vi "Keithley 6514 Block Read.vi"(0 "Resource In":refnum<visa-resource-name>, 1 "Check For SCPI Errors? (T)":bool=TRUE, 11 "error in (no error)":T1, 12 "Timeout (5000 msecs)":u32=5000) -> (4 "Resource Out (dupl)":refnum<visa-resource-name>, 6 "Num Meas":i32 min=0 max=2500, 8 "Test Data":sgl[][](array[numeric]) format="%^.4e", 10 "Data Elements":string, 15 "error out":T1)   [LabVIEW 2014, in "KE6514Driver.lvlib"]
doc: "This VI is used to perform a block read with the 6514. The VI will return the actual number of points that was read, the data format used for the data transfer, the data elements returned and the actual data which is stored in a LabVIEW array.\n\nNOTE: THIS VI WILL NOT EXECUTE CORRECTLY IF THE GPIB TIMEOUT FUNCTION IS NOT LONG ENOUGH. IF YOUR OPERATION TAKES LONGER THAN THE TIMEOUT PERIOD, INCORRECT OPERATION WILL OCCUR. THE VI SENDS OUT THE SCPI 'READ?' COMMAND. WHEN THIS COMMAND IS SENT OVER THE BUS, THE 24XX PERFORMS A SCPI 'INIT' FUNCTION WHICH INITIALIZES THE TRIGGERING AND BEGINS TAKING MEASUREMENTS. WHEN ALL MEASUREMENTS HAVE BEEN TAKEN, THE DATA IS RETURNED. AGAIN, IF THE TIMEOUT IS SMALLER THAN THE TIME IT TAKES TO COMPLETE THE MEASUREMENT OPERATIONS, INCORRECT RESULTS WILL OCCUR. IT IS RECOMMENDED TO SET THE TIMEOUT TO A LARGE VALUE TO PREVENT ERRORS.\n\nDEFAULTS: \nGPIB Address = 14\n\nMeasurements:\nReturned by instrument. Not user settable. 1 to 2500.\n\nData Format: \nReturned by instrument. Not user settable. Format returned is 'ASC' for ASCII and 'SRE' for Single Precision Real.\n\nData Elements:\nReturned by instrument. Not user settable. The order in which the elements are returned reflects the order in which each sample point is presented in the array. Main order is:\nREAD,TIME, STAT\n\nwhere:\nREAD = Reading\nTIME = Time Stamp\nSTAT = Status (Refer to Instrument Users manual to decode the status).\n\nTest Data:\nThis is an array where the sample data is placed after transfer over the bus. The order for which the data is presented appears in the 'Data Elements' indicator. Maximum number of data points returned is 2500."
uses:
  KE6514Driver.lvlib
panel:
  out "Max Num Bytes To Read For ASCII":i32
  out "Num Bytes To Read For Binary":i32
  out "Data Format":string
  # "NOTE: YOU MUST HAVE EXECUTED THE\n'BLOCK READ SETUP' VI AT LEAST ONCE\nPRIOR TO USING THIS VI."
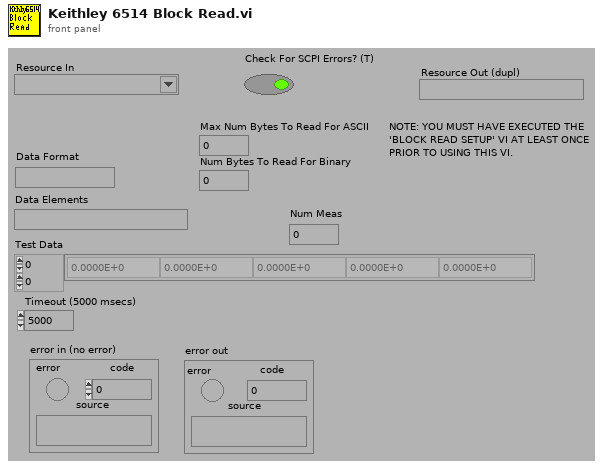
[diagram p1: front panel]
types:
  T1 = cluster{"error":bool, "code":i32, "source":string}
  T2 = enum16{"big-endian, network order", "native, host order", "little-endian"}
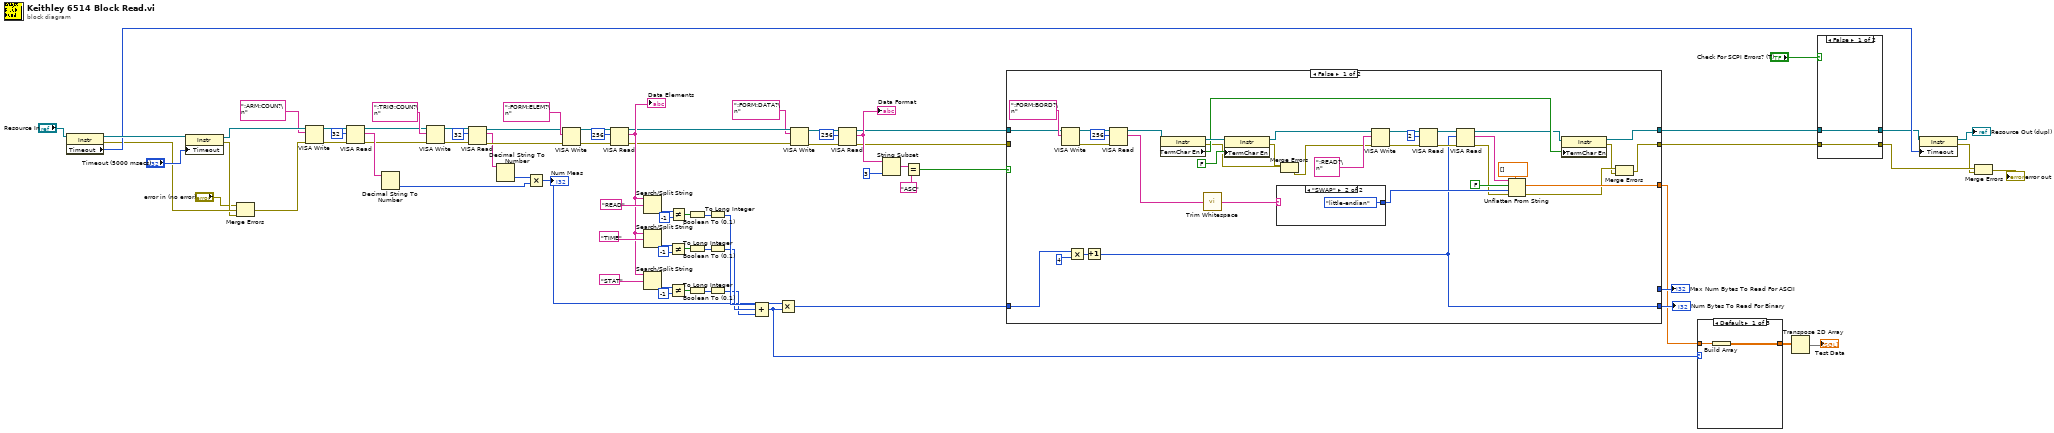
[diagram p0: block diagram]
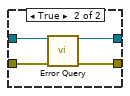
[diagram p2: hidden frame]
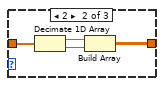
[diagram p3: hidden frame]
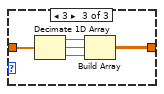
[diagram p4: hidden frame]
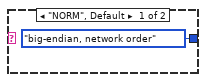
[diagram p5: hidden frame]
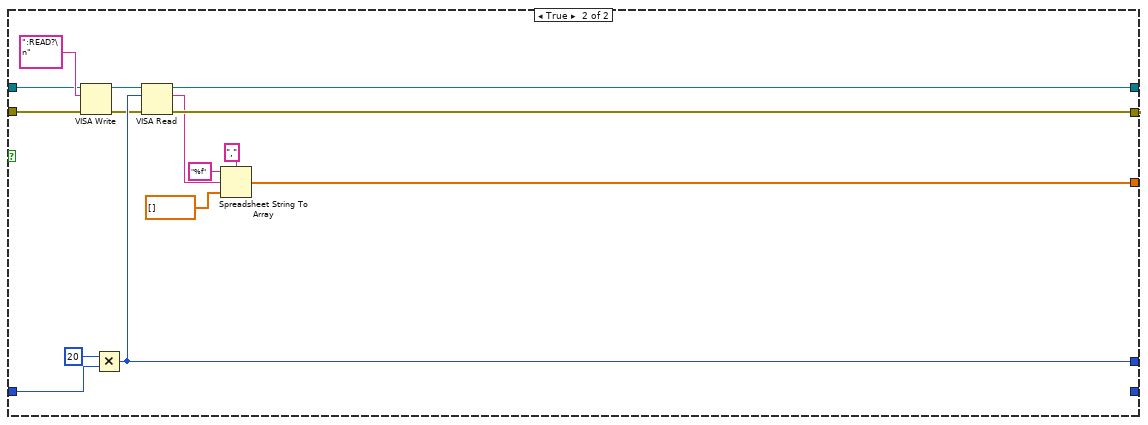
[diagram p6: hidden frame]
diagram:
  n1 = property class="Instr"(reference="Resource In") -> (reference out=w77:refnum<visa-resource-name>, error out=w4:errorcluster, "Timeout"=w13:u32)  [unwired: 1 in]
  n2 = property class="Instr"(reference=w77, "Timeout"="Timeout (5000 msecs)") -> (reference out=w75:refnum<visa-resource-name>, error out=w3:errorcluster)  [unwired: 1 in]
  n3 = Merge Errors("error in (no error)", w4, w3) -> (w1:errorcluster)
  n4 = VISA Write(VISA resource name=w75, write buffer=":ARM:COUN?\n", error in (no error)=w1) -> (VISA resource name out=w73:refnum<visa-resource-name>, error out=w71:errorcluster)  [unwired: 1 out]
  n5 = VISA Read(VISA resource name=w73, byte count=u32 32, error in (no error)=w71) -> (VISA resource name out=w65:refnum<visa-resource-name>, read buffer=w70:string, error out=w64:errorcluster)  [unwired: 1 out]
  n6 = Decimal String To Number(string=w70) -> (number=w63:i32)  [unwired: 2 in, 1 out]
  n7 = VISA Write(VISA resource name=w65, write buffer=":TRIG:COUN?\n", error in (no error)=w64) -> (VISA resource name out=w68:refnum<visa-resource-name>, error out=w66:errorcluster)  [unwired: 1 out]
  n8 = VISA Read(VISA resource name=w68, byte count=u32 32, error in (no error)=w66) -> (VISA resource name out=w58:refnum<visa-resource-name>, read buffer=w37:string, error out=w57:errorcluster)  [unwired: 1 out]
  n9 = Decimal String To Number(string=w37) -> (number=w36:i32)  [unwired: 2 in, 1 out]
  n10 = Multiply(x=w36, y=w63) -> (x*y=w24:i32)
  "Num Meas" <- w24
  n11 = VISA Write(VISA resource name=w58, write buffer=":FORM:ELEM?\n", error in (no error)=w57) -> (VISA resource name out=w61:refnum<visa-resource-name>, error out=w60:errorcluster)  [unwired: 1 out]
  n12 = VISA Read(VISA resource name=w61, byte count=u32 256, error in (no error)=w60) -> (VISA resource name out=w29:refnum<visa-resource-name>, read buffer=w38:string, error out=w27:errorcluster)  [unwired: 1 out]
  "Data Elements" <- w38
  n13 = Search/Split String(string=w38, search string/char (-)="TIME") -> (offset of match=w53:i32)  [unwired: 1 in, 2 out]
  n14 = Search/Split String(string=w38, search string/char (-)="STAT") -> (offset of match=w50:i32)  [unwired: 1 in, 2 out]
  n15 = Search/Split String(string=w38, search string/char (-)="READ") -> (offset of match=w55:i32)  [unwired: 1 in, 2 out]
  n16 = Not Equal?(x=w53, y=-1) -> (x != y?=w46:bool)
  n17 = Not Equal?(x=w50, y=-1) -> (x != y?=w45:bool)
  n18 = Not Equal?(x=w55, y=-1) -> (x != y?=w47:bool)
  n19 = Boolean To (0,1)(Boolean=w47) -> (0, 1=w44:i16)
  n20 = Boolean To (0,1)(Boolean=w46) -> (0, 1=w43:i16)
  n21 = Boolean To (0,1)(Boolean=w45) -> (0, 1=w42:i16)
  n22 = To Long Integer(number=w44) -> (32bit integer=w41:i32)
  n23 = To Long Integer(number=w43) -> (32bit integer=w40:i32)
  n24 = To Long Integer(number=w42) -> (32bit integer=w39:i32)
  n25 = Compound Arithmetic op=ADD(w41, w40, w39) -> (w20:i32)
  n26 = Multiply(x=w24, y=w20) -> (x*y=w23:i32)
  n27 = VISA Write(VISA resource name=w29, write buffer=":FORM:DATA?\n", error in (no error)=w27) -> (VISA resource name out=w31:refnum<visa-resource-name>, error out=w30:errorcluster)  [unwired: 1 out]
  n28 = VISA Read(VISA resource name=w31, byte count=u32 256, error in (no error)=w30) -> (VISA resource name out=w6:refnum<visa-resource-name>, read buffer=w26:string, error out=w5:errorcluster)  [unwired: 1 out]
  "Data Format" <- w26
  n29 = String Subset(string=w26, length (rest)=3) -> (substring=w33:string)  [unwired: 1 in]
  n30 = Equal?(x=w33, y="ASC") -> (x = y?=w25:bool)
  n31 = case shown="False" w25 {
    tunnel: w23 -> [w85 w123]
    tunnel: [w78 w130] -> w14
    tunnel: w6 -> [w87 w119]
    tunnel: [w101 w129] -> w15
    tunnel: [w88 w124] -> w19
    tunnel: [_ w121] -> w22
    tunnel: [w84 _] -> w21
    tunnel: w5 -> [_ w118]
    frame False {
      n32 = VISA Write(VISA resource name=w87, write buffer=":FORM:BORD?\n") -> (VISA resource name out=w99:refnum<visa-resource-name>, error out=w98:errorcluster)  [unwired: 1 in, 1 out]
      n33 = Multiply(x=w85, y=4) -> (x*y=w113:i32)
      n34 = Increment(x=w113) -> (x+1=w84:i32)
      n35 = VISA Read(VISA resource name=w99, byte count=u32 256, error in (no error)=w98) -> (VISA resource name out=w96:refnum<visa-resource-name>, read buffer=w93:string)  [unwired: 2 out]
      n36 = property class="Instr"(reference=w96) -> (reference out=w112:refnum<visa-resource-name>, error out=w83:errorcluster, "TermChar En"=w102:bool)  [unwired: 1 in]
      n37 = call <vilib>:"Trim Whitespace.vi"("string"=w93) -> ("trimmed string"=w90:string)  [unwired: 1 in]
      n38 = property class="Instr"(reference=w112, "TermChar En"=FALSE ("Message Based Settings:Termination Character Enable")) -> (reference out=w107:refnum<visa-resource-name>, error out=w82:errorcluster)  [unwired: 1 in]
      n39 = case shown="\"SWAP\"" w90 {
        tunnel: [T2."big-endian, network order" ("byte order (0:big-endian, network order)") T2."little-endian" ("byte order (0:big-endian, network order)")] -> w92
        frame "NORM", Default {
        }
        frame "SWAP" {
        }
      }
      n40 = Merge Errors(w83, w82) -> (w81:errorcluster)
      n41 = VISA Write(VISA resource name=w107, write buffer=":READ?\n", error in (no error)=w81) -> (VISA resource name out=w109:refnum<visa-resource-name>, error out=w108:errorcluster)  [unwired: 1 out]
      n42 = VISA Read(VISA resource name=w109, byte count=u32 2, error in (no error)=w108) -> (VISA resource name out=w104:refnum<visa-resource-name>, error out=w105:errorcluster)  [unwired: 2 out]
      n43 = VISA Read(VISA resource name=w104, byte count=w84, error in (no error)=w105) -> (VISA resource name out=w89:refnum<visa-resource-name>, read buffer=w95:string, error out=w91:errorcluster)  [unwired: 1 out]
      n44 = Unflatten From String(type=sgl[] [], binary string=w95, data includes array or string size? (T)=FALSE, byte order (0:big-endian, network order)=w92, error in (no error)=w91) -> (value=w88:sgl[], error out=w80:errorcluster)  [unwired: 1 out]
      n45 = property class="Instr"(reference=w89, "TermChar En"=w102) -> (reference out=w101:refnum<visa-resource-name>, error out=w79:errorcluster)  [unwired: 1 in]
      n46 = Merge Errors(w80, w79) -> (w78:errorcluster)
    }
    frame True {
      n47 = VISA Write(VISA resource name=w119, write buffer=":READ?\n", error in (no error)=w118) -> (VISA resource name out=w116:refnum<visa-resource-name>, error out=w117:errorcluster)  [unwired: 1 out]
      n48 = Multiply(x=20, y=w123) -> (x*y=w121:i32)
      n49 = VISA Read(VISA resource name=w116, byte count=w121, error in (no error)=w117) -> (VISA resource name out=w129:refnum<visa-resource-name>, read buffer=w128:string, error out=w130:errorcluster)  [unwired: 1 out]
      n50 = Spreadsheet String To Array(delimiter (Tab)=",", format string="%f", spreadsheet string=w128, array type (2D Dbl)=sgl[] []) -> (array=w124:sgl[])
    }
  }
  "Num Bytes To Read For Binary" <- w21
  "Max Num Bytes To Read For ASCII" <- w22
  n51 = case shown="Default" w20 {
    tunnel: [w131 w133 w137] -> w18
    tunnel: w19 -> [w132 w136 w141]
    frame Default {
      n52 = Build Array(w132) -> (w131:sgl[][])
    }
    frame 2 {
      n53 = Decimate 1D Array(w136) -> (w135:sgl[], w134:sgl[])
      n54 = Build Array(w135, w134) -> (w133:sgl[][])
    }
    frame 3 {
      n55 = Decimate 1D Array(w141) -> (w140:sgl[], w139:sgl[], w138:sgl[])
      n56 = Build Array(w140, w139, w138) -> (w137:sgl[][])
    }
  }
  n57 = Transpose 2D Array(2D array=w18) -> (transposed array=→"Test Data":sgl[][])
  n58 = case shown="False" "Check For SCPI Errors? (T)" {
    tunnel: w15 -> [w143 w147]
    tunnel: w14 -> [w142 w146]
    tunnel: [w143 w145] -> w12
    tunnel: [w142 w144] -> w11
    frame False {
    }
    frame True {
      n59 = call "Error Query.vi"("VISA Resource In"=w147, "error in (no error)"=w146) -> ("VISA Resource Out (dupl)"=w145:refnum<visa-resource-name>, "error out"=w144:errorcluster)  [unwired: 10 in, 2 out]
    }
  }
  n60 = property class="Instr"(reference=w12, "Timeout"=w13) -> (reference out=→"Resource Out (dupl)":refnum<visa-resource-name>, error out=w10:errorcluster)  [unwired: 1 in]
  n61 = Merge Errors(w11, w10) -> (→"error out":errorcluster)
